vi "ShowError.vi"(10 "String":string, 11 "ErrorStatus Refnum in":refnum<k24>) -> ()   [LabVIEW 2023]
uses:
  C:/Program Files/National Instruments/LabVIEW 2025/MechEyeApiNet.dll
  Program Files/National Instruments/LabVIEW 2025/MechEyeApiNet.dll
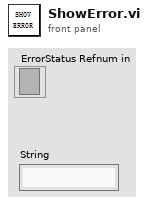
[diagram p1: front panel]
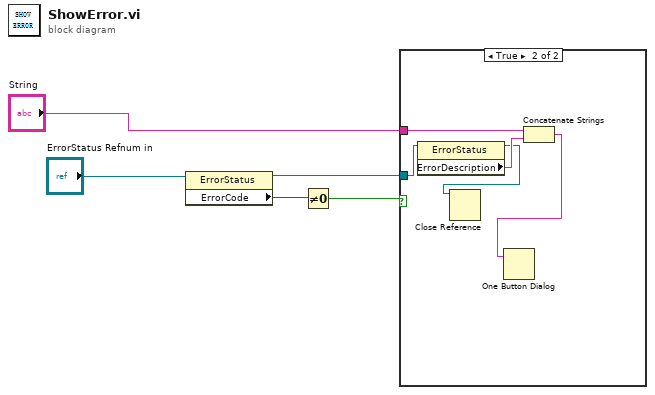
[diagram p0: block diagram]
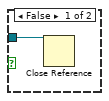
[diagram p2: hidden frame]
diagram:
  n1 = property class="ErrorStatus"(reference="ErrorStatus Refnum in") -> (reference out=w4:refnum<k24>, "ErrorCode"=w2:i32)  [unwired: 1 in, 1 out]
  n2 = Not Equal To 0?(x=w2) -> (x != 0?=w3:bool)
  n3 = case shown="True" w3 {
    tunnel: w4 -> [w6 w11]
    tunnel: "String" -> [_ w10]
    frame False {
      n4 = Close Reference(reference=w6) -> ()  [unwired: 1 in, 1 out]
    }
    frame True {
      n5 = property class="ErrorStatus"(reference=w11) -> (reference out=w7:refnum<k24>, "ErrorDescription"=w9:string)  [unwired: 1 in, 1 out]
      n6 = Close Reference(reference=w7) -> ()  [unwired: 1 in, 1 out]
      n7 = Concatenate Strings(w10, w9) -> (w8:string)
      n8 = One Button Dialog(message=w8) -> ()  [unwired: 1 in, 1 out]
    }
  }
